vi "Find Tests.vi"(8 "error in (no error)":errorcluster, 10 "File Paths":path[](array[path]), 11 "LUnit Test Suite":refnum<class "LUnit Test Suite.lvclass">) -> (0 "error out":errorcluster, 3 "LUnit Test Suite":refnum<class "LUnit Test Suite.lvclass">)   [LabVIEW 2020, in "Test Finder.lvclass"]
uses:
  Test Finder.lvclass
  Test Finder.lvclass/Test Finder.ctl
  LUnit Test Suite.lvclass
  C:/git/astemes-lunit/source/LUnit Test Suite.lvclass
  C:/git/astemes-lunit/source/Runnable.lvclass
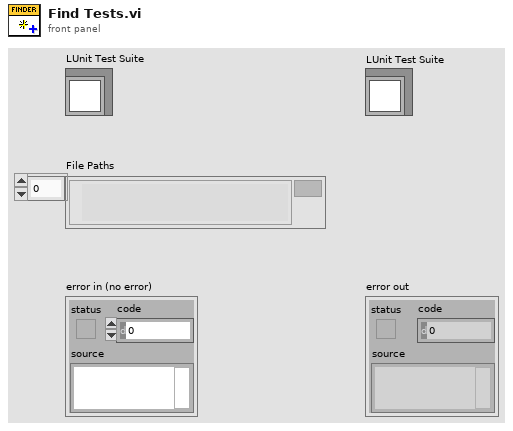
[diagram p1: front panel]
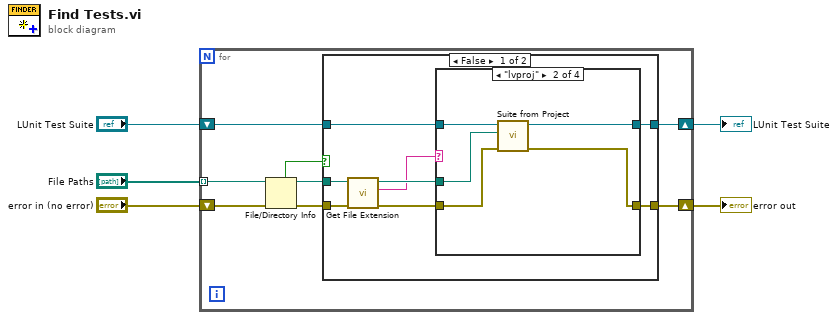
[diagram p0: block diagram]
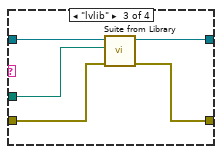
[diagram p3: hidden frame]
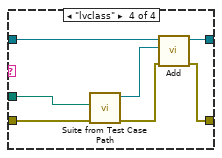
[diagram p4: hidden frame]
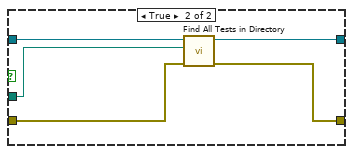
[diagram p5: hidden frame]
diagram:
  n1 = for {
    tunnel: "File Paths" -> [w8] mode=indexing
    shift-right: [w10] -> w4
    shift-left: "error in (no error)" -> [w13]
    shift-right: [w11] -> w3
    shift-left: "LUnit Test Suite" -> [w12]
    n2 = File/Directory Info(path=w8, error in=w13) -> (path out=w7:path, directory=w6:bool, error out=w9:errorcluster)  [unwired: 4 out]
    n3 = case shown="False" w6 {
      tunnel: w12 -> [w21 w45]
      tunnel: [w20 w44] -> w11
      tunnel: [w19 w43] -> w10
      tunnel: w9 -> [w15 w42]
      tunnel: w7 -> [w14 w41]
      frame False {
        n4 = call <vilib>:"Get File Extension.vi"("error in (no error)"=w15, "file"=w14) -> ("error out"=w18:errorcluster, "lowercase file extension"=w16:string, "dup file"=w17:path)  [unwired: 5 in, 2 out]
        n5 = case shown="\"lvproj\"" w16 {
          tunnel: w21 -> [w23 w24 w29 w36]
          tunnel: [w23 w25 w30 w38] -> w20
          tunnel: [w22 w28 w33 w34] -> w19
          tunnel: w18 -> [w22 w27 w32 w40]
          tunnel: w17 -> [_ w26 w31 w39]
          frame Default {
          }
          frame "lvproj" {
            n6 = call "Suite from Project.vi"("error in (no error)"=w27, "Project Path"=w26, "LUnit Test Suite In"=w24) -> ("error out"=w28:errorcluster, "LUnit Test Suite Out"=w25:refnum<class "LUnit Test Suite.lvclass">)  [unwired: 7 in]
          }
          frame "lvlib" {
            n7 = call "Suite from Library.vi"("error in (no error)"=w32, "Library Path"=w31, "LUnit Test Suite In"=w29) -> ("error out"=w33:errorcluster, "LUnit Test Suite Out"=w30:refnum<class "LUnit Test Suite.lvclass">)  [unwired: 7 in]
          }
          frame "lvclass" {
            n8 = call "Suite from Test Case Path.vi"("error in (no error)"=w40, "Test Case"=w39) -> ("error out"=w35:errorcluster, "LUnit Test Suite Out"=w37:refnum<class "LUnit Test Suite.lvclass">)  [unwired: 8 in]
            n9 = call "Add.vi"("error in (no error)"=w35, "Runnable"=w37, "LUnit Test Suite In"=w36) -> ("error out"=w34:errorcluster, "LUnit Test Suite Out"=w38:refnum<class "LUnit Test Suite.lvclass">)  [unwired: 7 in]
          }
        }
      }
      frame True {
        n10 = call "Find All Tests in Directory.vi"("error in (no error)"=w42, "Directory Path"=w41, "LUnit Test Suite In"=w45) -> ("error out"=w43:errorcluster, "LUnit Test Suite out"=w44:refnum<class "LUnit Test Suite.lvclass">)  [unwired: 7 in]
      }
    }
  }
  "error out" <- w4
  "LUnit Test Suite" <- w3
